vi "To PCM task.vi"(10 "task":u64) -> (2 "PCM task":T1)   [LabVIEW 2022 SP3, in "DAAG task conversion.lvlib"]
uses:
  <vilib>/PDM Acquisition Toolkit/host/Classes/Tasks/PCM Input/Controls/DVR PCM Input Task.ctl
  <vilib>/PDM Acquisition Toolkit/host/Classes/Tasks/PCM Input/PCM Input Task.lvclass
  DAAG task conversion.lvlib
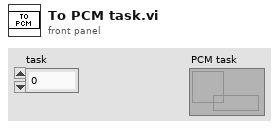
[diagram p1: front panel]
types:
  T1 = typedef "PDM Acquisition Class Library.lvlib/PCM Input Task.lvclass/DVR PCM Input Task.ctl" = refnum<data-value>
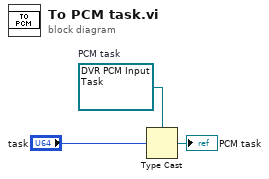
[diagram p0: block diagram]
diagram:
  w3 = T1 refnum  # PCM task
  n1 = Type Cast(type=w3, x="task") -> (*(type *) &x=→"PCM task":T1)
